vi "Actor Core.vi"(8 "error in":errorcluster, 11 "Customer in":refnum<class "Customer.lvclass">) -> (0 "error out":errorcluster, 3 "Actor out":refnum<class "Actor.lvclass">)   [LabVIEW 2023, in "Customer.lvlib" / "Customer.lvclass"]
doc: "(<B>Filename</B>: Actor Framework.lvlib:Actor.lvclass:Actor Core.vi)\n\nReceives messages to the actor, reacts to them, and initiates any error handling that may shut the actor down.\n\nDescendant classes may override this VI to append parallel tasks for the actor to complete while it handles messages. Overrides use the Call Parent Method node."
uses:
  Customer.lvclass
  c:/dev/_r/4/eng/lv-core/lvpostprocessingd/lv_mc_x86_64/dist_i386/examples/Design Patterns/Actor Framework/Classes/Person/Person.lvclass
  c:/dev/_r/4/eng/lv-core/lvpostprocessingd/lv_mc_x86_64/dist_i386/vi.lib/ActorFramework/Actor/Actor.lvclass
  <vilib>/ActorFramework/Actor/Actor.lvclass
  Beverages/TypeDefs/Drink Type.ctl
  Beverages/TypeDefs/Options.ctl
  Person/Person.lvclass/Person.ctl
  Customer.lvclass/Customer.ctl
  <vilib>/ActorFramework/Actor/Actor.lvclass/Actor.ctl
  <vilib>/ActorFramework/Message Enqueuer/Message Enqueuer.lvclass/Message Enqueuer.ctl
  Person Messages/Show or Hide Front Panel Msg/Show or Hide Front Panel Msg.lvclass/Show or Hide Front Panel Msg.ctl
  Work Dispatcher Messages/Add Task Msg/Add Task Msg.lvclass/Add Task Msg.ctl
  <vilib>/ActorFramework/Stop Msg/Stop Msg.lvclass
  c:/dev/_r/4/eng/lv-core/lvpostprocessingd/lv_mc_x86_64/dist_i386/vi.lib/ActorFramework/Message/Message.lvclass
  <vilib>/ActorFramework/Message Enqueuer/Init from Existing Queue.vi
  <vilib>/ActorFramework/Message Enqueuer/Enqueue.vi
  Person Messages/Show or Hide Front Panel Msg/Show or Hide Front Panel Msg.lvclass
  Work Dispatcher Messages/Add Task Msg/Add Task Msg.lvclass
  <vilib>/ActorFramework/Message Priority Queue/Priority Enqueue.vi
  <vilib>/ActorFramework/Message Enqueuer/Message Enqueuer.lvclass
  Person/Person.lvclass
  Order/Order.lvclass
  Beverages/Beverage/Beverage.lvclass
panel:
  in  "Customer Info":string="Received %d of %d"
  in  "Received":string="Received %d of %d"
  out "All Items Received":bool
  out "Order in progress":bool
  out "Items Ordered":i32
  out "Items Received":i32
  in  "Items Picked Up":string
  out "Price":dbl
  out "Order Number":dbl
  in  "Reset Order":bool
  in  "Make Order":bool
  in  "Order":cluster{"Drink type":T1, "Options":T2[]}[](array[cluster])
  out "Name":string="<name>"
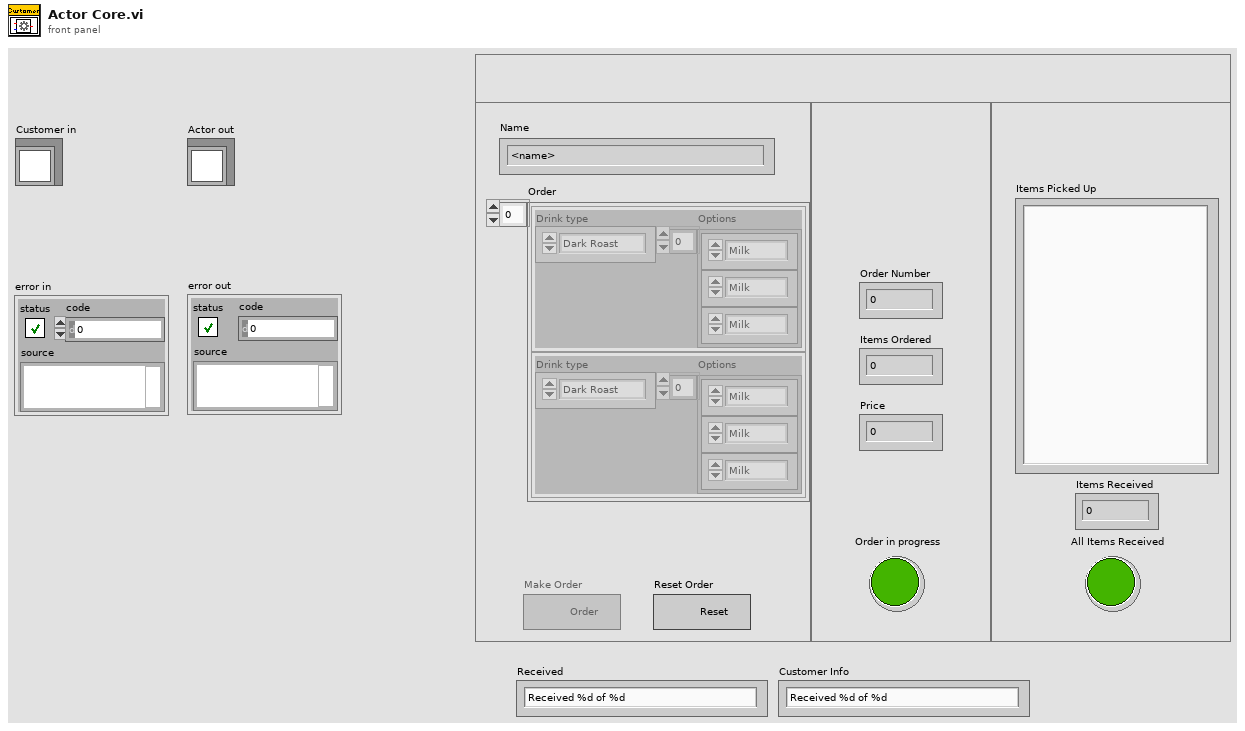
[diagram p1: front panel]
types:
  T1 = typedef "Beverage.lvclass/Drink Type.ctl" = enum16{"Dark Roast", "Decaf", "Espresso", "House Blend"}
  T2 = typedef "Beverage.lvclass/Options.ctl" = enum16{"<None>", "Milk", "Mocha", "Soy", "Whip"}
  T3 = enum8{"Enabled", "Disabled", "Disabled and Grayed Out"}
  T4 = cluster{"Item":refnum<user-event>, "Order #":refnum<user-event>, "Stop":refnum<user-event>}
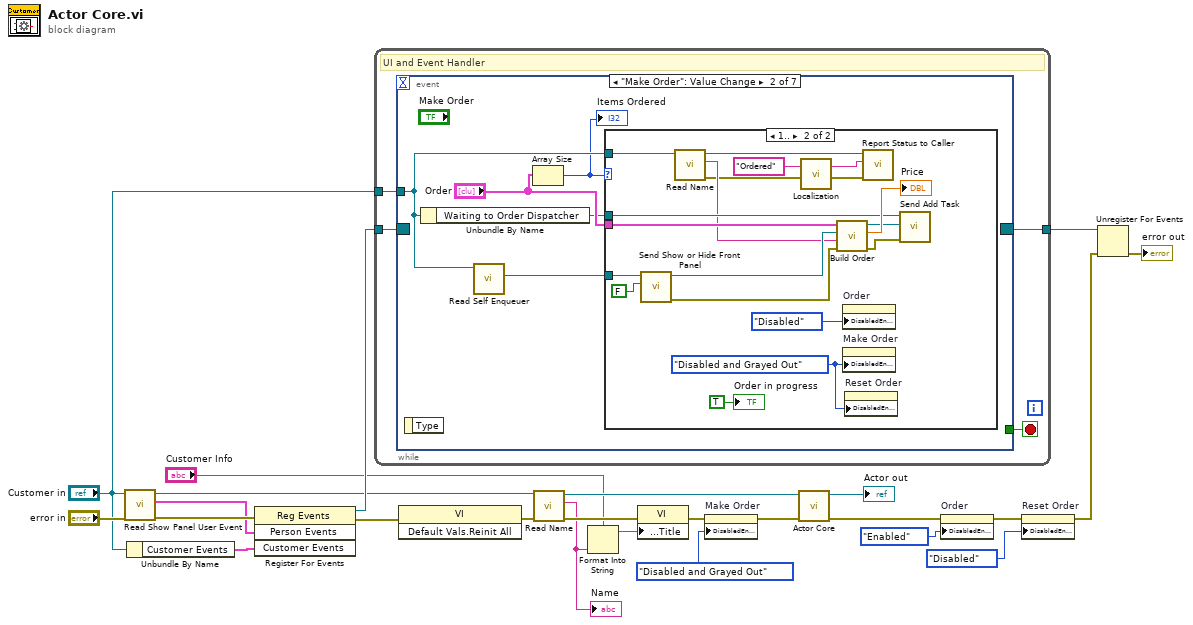
[diagram p0: block diagram]
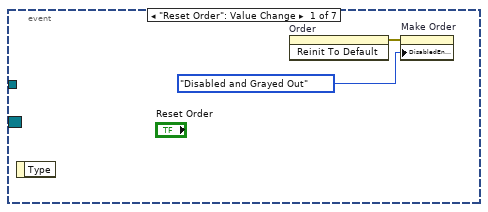
[diagram p2: hidden frame]
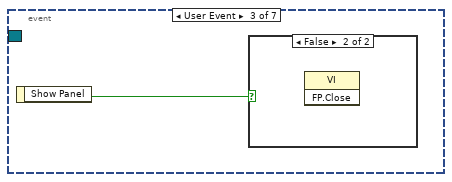
[diagram p4: hidden frame]
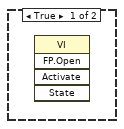
[diagram p5: hidden frame]
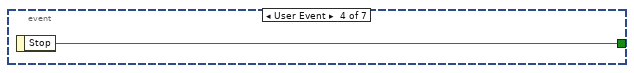
[diagram p6: hidden frame]
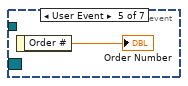
[diagram p7: hidden frame]
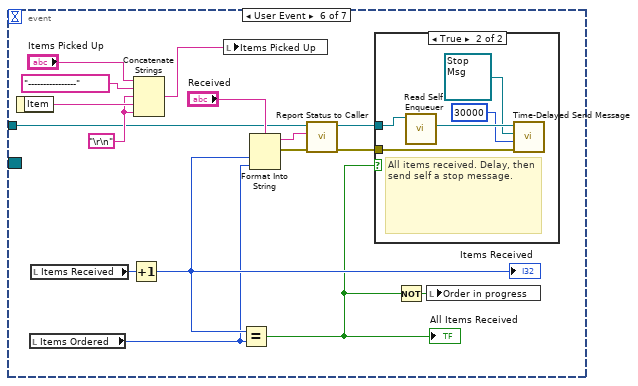
[diagram p8: hidden frame]
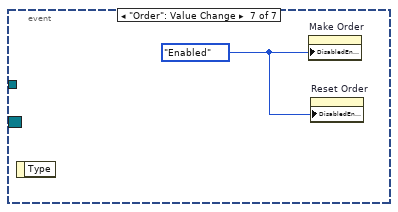
[diagram p10: hidden frame]
diagram:
  n1 = call "Read Show Panel User Event.vi"("error in (no error)"="error in", "Person in"="Customer in") -> ("error out"=w6:errorcluster, "Person Events"=w5:cluster{"Show Panel":refnum<user-event>}, "Person out"=w7:refnum<class "Customer.lvclass">)  [unwired: 7 in]
  n2 = Unbundle By Name("Customer in") -> ("Customer Events"=w4:T4)
  n3 = register-events(error in=w6, w5, w4) -> (reference out=w23:refnum<event-registration>, error out=w15:errorcluster)  [unwired: 1 in]
  n4 = while {
    tunnel: w23 -> [w28]
    tunnel: "Customer in" -> [w27]
    tunnel: [w26] -> w12
    stop <- w29 stop-if-true
    # "UI and Event Handler"
    n5 = event shown="[1] \"Make Order\": Value Change" {
      selector: w28 -> [_ _ _ _ _ _ _]
      dyn-events: [_ _ _ _ _ _ _] -> w26
      timeout: _ -> [_ _ _ _ _ _ _]
      tunnel: [_ _ _ w56 _ _ _] -> w29
      tunnel: w27 -> [_ w33 _ _ _ w61 _]
      event "Reset Order": Value Change {
        n6 = event-data() -> ()  [unwired: 1 in, 1 out]
        n7 = invoke on="Order" class="Arr (strict)" method="Reinit To Default"() -> (error out=w30:errorcluster)  [unwired: 3 in, 2 out]
        n8 = property on="Make Order" class="Bool"(error in=w30, "DisabledEnum"=T3."Disabled and Grayed Out" ("Disabled")) -> ()  [unwired: 1 in, 2 out]
      }
      event "Make Order": Value Change {
        n9 = event-data() -> ()  [unwired: 1 in, 1 out]
        n10 = Unbundle By Name(w33) -> ("Waiting to Order Dispatcher"=w35:refnum<class "Message Enqueuer.lvclass">)
        n11 = call <vilib>:"Read Self Enqueuer.vi"("Actor"=w33) -> ("Self Enqueuer"=w34:refnum<class "Message Enqueuer.lvclass">)  [unwired: 10 in]
        n12 = Array Size(array="Order") -> (size(s)=w32:i32)
        "Items Ordered" <- w32
        n13 = case shown="1.." w32 {
          tunnel: "Order" -> [_ w51]
          tunnel: w35 -> [_ w50]
          tunnel: w34 -> [_ w46]
          tunnel: w33 -> [_ w44]
          frame 0, Default {
            # "Do nothing if the order contains no items"
          }
          frame 1.. {
            w48 = T3."Disabled and Grayed Out" ("Disabled")
            n14 = call "Send Show or Hide Front Panel.vi"("Show Front Panel?"=FALSE, "Message Enqueuer"=w46) -> ("error out"=w40:errorcluster, "Message Enqueuer out"=w45:refnum<class "Message Enqueuer.lvclass">)  [unwired: 8 in]
            n15 = call-dynamic "Read Name.vi"("Person in"=w44) -> ("error out"=w41:errorcluster, "Name"=w42:string, "Person out"=w43:refnum<class "Customer.lvclass">)  [unwired: 8 in]
            n16 = call "Localization.vi"("untranslated"="Ordered" ("Status")) -> ("translated"=w38:string)  [unwired: 2 in]
            n17 = call "Build Order.vi"("error in (no error)"=w40, "Name"=w42, "Customer"=w45, "Order"=w51) -> ("error out"=w53:errorcluster, "Cost"=→"Price":dbl, "Order Out"=w52:refnum<class "Order.lvclass">)  [unwired: 5 in]
            n18 = property on="Order" class="Arr (strict)"("DisabledEnum"=T3."Disabled" ("Disabled")) -> ()  [unwired: 2 in, 2 out]
            n19 = property on="Make Order" class="Bool"("DisabledEnum"=w48) -> ()  [unwired: 2 in, 2 out]
            n20 = property on="Reset Order" class="Bool"("DisabledEnum"=w48) -> ()  [unwired: 2 in, 2 out]
            n21 = call-dynamic "Report Status to Caller.vi"("error in"=w41, "Status"=w38, "Customer in"=w43) -> ()  [unwired: 7 in, 2 out]
            n22 = call "Send Add Task.vi"("error in (no error)"=w53, "Task"=w52, "Message Enqueuer"=w50) -> ()  [unwired: 7 in, 2 out]
            "Order in progress" <- TRUE ("Order in progress")
          }
        }
      }
      event User Event {
        n23 = event-data() -> ("Show Panel"=w55:bool)  [unwired: 1 in]
        n24 = case shown="False" w55 {
          frame True {
            n25 = invoke on="Invoke Node" class="VI" method="FP.Open"() -> ()  [unwired: 5 in, 5 out]
          }
          frame False {
            n26 = invoke on="Invoke Node" class="VI" method="FP.Close"() -> ()  [unwired: 3 in, 3 out]
          }
        }
      }
      event User Event {
        n27 = event-data() -> ("Stop"=w56:bool)  [unwired: 1 in]
      }
      event User Event {
        n28 = event-data() -> ("Order #"=→"Order Number":dbl)  [unwired: 1 in]
      }
      event User Event {
        w69 = "\r\n" ("End of Line Constant")
        n29 = event-data() -> ("Item"=w71:string)  [unwired: 1 in]
        n30 = local read "Items Ordered"() -> (w65:i32)
        n31 = local read "Items Received"() -> (w60:i32)
        n32 = Increment(x=w60) -> (x+1=w66:i32)
        "Items Received" <- w66
        n33 = Concatenate Strings("Items Picked Up", "----------------" ("string"), w69, w71, w69) -> (w72:string)
        n34 = local write "Items Picked Up"(w72) -> ()
        n35 = Equal?(x=w66, y=w65) -> (x = y?=w62:bool)
        "All Items Received" <- w62
        n36 = Format Into String(format string="Received", w66, w65) -> (resulting string=w64:string, error out=w63:errorcluster)  [unwired: 2 in]
        n37 = call-dynamic "Report Status to Caller.vi"("error in"=w63, "Status"=w64, "Customer in"=w61) -> ("error out"=w58:errorcluster, "Customer out"=w59:refnum<class "Customer.lvclass">)  [unwired: 7 in]
        n38 = case shown="True" w62 {
          tunnel: w59 -> [_ w75]
          tunnel: w58 -> [_ w74]
          frame False {
          }
          frame True {
            # "All items received. Delay, then send self a stop message."
            n39 = call <vilib>:"Read Self Enqueuer.vi"("Actor"=w75) -> ("Self Enqueuer"=w78:refnum<class "Message Enqueuer.lvclass">)  [unwired: 10 in]
            n40 = call <vilib>:"Time-Delayed Send Message.vi"("error in (no error)"=w74, "Milliseconds To Wait"=30000, "Message"=refnum<class "Stop Msg.lvclass"> refnum ("Actor Framework.lvlib:Stop Msg"), "Message Enqueuer"=w78) -> ()  [unwired: 6 in, 2 out]
          }
        }
        n41 = Not(x=w62) -> (.not. x?=w68:bool)
        n42 = local write "Order in progress"(w68) -> ()
      }
      event "Order": Value Change {
        w79 = T3."Enabled" ("Disabled")
        n43 = event-data() -> ()  [unwired: 1 in, 1 out]
        n44 = property on="Make Order" class="Bool"("DisabledEnum"=w79) -> ()  [unwired: 2 in, 2 out]
        n45 = property on="Reset Order" class="Bool"("DisabledEnum"=w79) -> ()  [unwired: 2 in, 2 out]
      }
    }
  }
  n46 = invoke on="Invoke Node" class="VI" method="Default Vals.Reinit All"(error in=w15) -> (error out=w18:errorcluster)  [unwired: 2 in, 2 out]
  n47 = call-dynamic "Read Name.vi"("error in (no error)"=w18, "Person in"=w7) -> ("error out"=w13:errorcluster, "Name"=w3:string, "Person out"=w19:refnum<class "Customer.lvclass">)  [unwired: 7 in]
  "Name" <- w3
  n48 = Format Into String(format string="Customer Info", w3) -> (resulting string=w2:string)  [unwired: 2 in, 1 out]
  n49 = property on="Property Node" class="VI"(error in=w13, "Front Panel.Title"=w2) -> (error out=w14:errorcluster)  [unwired: 1 in, 1 out]
  n50 = property on="Make Order" class="Bool"(error in=w14, "DisabledEnum"=T3."Disabled and Grayed Out" ("Disabled")) -> (error out=w24:errorcluster)  [unwired: 1 in, 1 out]
  n51 = call-parent "Actor Core.vi"("error in"=w24, "Actor in"=w19) -> ("error out"=w22:errorcluster, "Actor out"=→"Actor out":refnum<class "Actor.lvclass">)  [unwired: 8 in]
  n52 = property on="Order" class="Arr (strict)"(error in=w22, "DisabledEnum"=T3."Enabled" ("Disabled")) -> (error out=w17:errorcluster)  [unwired: 1 in, 1 out]
  n53 = property on="Reset Order" class="Bool"(error in=w17, "DisabledEnum"=T3."Disabled" ("Disabled")) -> (error out=w11:errorcluster)  [unwired: 1 in, 1 out]
  n54 = Unregister For Events(event registration refnum=w12, error in=w11) -> (error out=→"error out":errorcluster)
